vi "Player Info.vi"(11 "Template in":refnum<class "Demo.lvclass">) -> (0 "Defeat Speech":string, 1 "Victory Speech":string, 2 "Name":string, 3 "Template out":refnum<class "Demo.lvclass">)   [LabVIEW 2015, in "Demo.lvclass"]
uses:
  Demo.lvclass
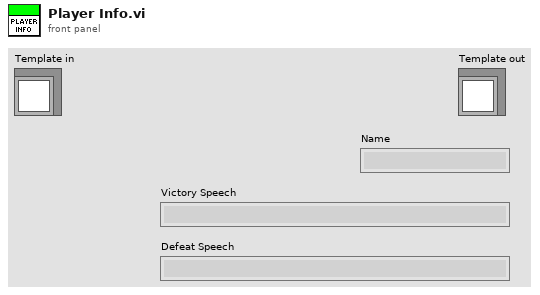
[diagram p1: front panel]
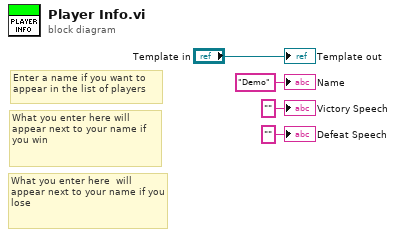
[diagram p0: block diagram]
diagram:
  # "What you enter here  will appear next to your name if you lose"
  # "What you enter here will appear next to your name if you win"
  # "Enter a name if you want to appear in the list of players"
  "Template out" <- "Template in"
  "Name" <- "Demo" ("Name")
  "Victory Speech" <- "" ("Victory Speech")
  "Defeat Speech" <- "" ("Defeat Speech")
